vi "Test Control Panel(Blake).vi"() -> ()   [LabVIEW 2017, in "Synapse CCD.lvclass"]
uses:
  Synapse CCD.lvclass
  Areas.ctl
  <vilib>/Utility/error.llb/DialogType.ctl
  Synapse CCD.lvclass/Synapse CCD.ctl
  Spectrometer Triax 550/JY-SPEX-TRIAX/controls.llb/Slits.ctl
  Global/GPIB Numbers.vi
  Spectrometer Triax 550/JY-SPEX-TRIAX/JY-SPEX-TRIAX.lvlib
panel:
  out "laser Pulse":dbl[unit]
  in  "estimate laser Pulse?":bool
  in  "error in (no error)":errorcluster
  out "CCD \nInitialized":bool
  out "JYCCDLib.IJYCCDReqd 1":refnum<k7>
  out "Spectrometer \nInitialized":bool
  in  "File Name":path
  out "error out":errorcluster
  in  "Go to start\nof raster scan":bool
  in  "Raster explanation":bool
  in  "Repeat Capture":bool
  in  "Export\nPlot":bool
  in  "Take Spectrum":bool
  in  "Set CCD":bool
  in  "Set Grating":bool
  in  "Copy Actual to Set":bool
  in  "Populate Fields with Member Data":bool
  in  "Bin width (pixels)":i32=1 min=1 max=1024 step=1
  in  "Number of CCD bins to use each snapshot":i32=1 min=1 max=1024 step=1
  in  "Raster Scan":bool
  in  "Cosmic Ray\nRemoval?":bool
  in  "# to Average":u32=1
  in  "Averaging?":bool
  in  "Time Between Acq. (ms)":u32
  in  "Dark Subtract?":bool
  out "Status":string
  out "Max slit resolution":dbl[unit]
  out "Warning: counts \nwent too high!":bool
  out "Resolution\n(nm/pixel)":dbl[unit] format="%#_3g"
  out "where am i?":string
  out "Total possible CCD bins":dbl=20.48
  out "Cosmic Ray Locations":string
  out "Bin width (nm)\n(scan resolution)":dbl[unit]=3.7e-11
  in  "Start":dbl[unit]
  in  "End":dbl[unit]
  in  "Exit Slit":dbl[unit]
  in  "Entrance Slit":dbl[unit]
  out "Min":dbl[unit]
  out "Max":dbl[unit]
  in  "Center Wavelength":dbl[unit]
  in  "Grating":u16(ring) items=["1200 lines/mm - 500 nm Blaze", "1200 lines/mm - 750 nm Blaze", "600 lines/mm - 1000 nm Blaze"]
  in  "GAIN":u16(ring) caption="Device Name" items=["High Light", "Best Dynamic", "High Sensitivity"]
  in  "ADC":u16(ring) caption="Device Name" items=["   20 kHz", "1 MHz", "1 MHz Ultra"]
  in  "Integration time":dbl[unit]=0.01
  in  "stop":bool
  in  "image mode":bool
  out "Spectrum":cluster{"Ramp Pattern":dbl[], "X array":dbl[]}[](graph)
  out "UnProcessed Spectra":T1(graph)
  out "Max value of last snapshot":i32
  out "populate fields with member data: CCD private data":T3={"JYCCDLib.IJYCCDReqd"=refnum, "JYMONOLib.IJYMonoReqd"=refnum, "Integration time"=0.01, "ADC"=0, "GAIN"=0, "Areas"=[[1, 1, 1, 1024, 256, 1, 256]], "Most Recent Data Object"=refnum, "Mono Properties"={"Grating"=0, "Center Wavelength"=0.0, "Entrance Slit"=0.0, "Exit Slit"=0.0}, "Coverage"={"Max"=0.0, "Min"=0.0}, "Multi-Acquisitions"={"Dark Subtract?"=FALSE, "Averaging?"=FALSE, "Cosmic Ray Removal?"=FALSE, "# to Average"=0, "Time Between Acq."=0, "Acquisitions Control Array"=[TRUE], "Raw Data"=[], "Processed Data"=[], "Array of Wavelengths"=[]}, "Raster Scan"={"Raster Scan?"=FALSE, "Start"=0.0, "End"=0.0, "Bin width (pixels)"=1, "Bin width (nm)\n(scan resolution)"=3.7e-11, "Number of CCD bins to use each snapshot"=1, "Total possible CCD bins"=20.48, "Warning: counts \nwent too high!"=FALSE}} {"Raster Scan"."Number of CCD bins to use each snapshot" min=1 max=1024 step=1; "Raster Scan"."Bin width (pixels)" min=1 max=1024 step=1; "Mono Properties"."Grating" items=["1200 lines/mm - 500 nm Blaze", "1200 lines/mm - 750 nm Blaze", "600 lines/mm - 1000 nm Blaze"]; "GAIN" items=["High Light", "Best Dynamic", "High Sensitivity"]; "ADC" items=["   20 kHz", "1 MHz", "1 MHz Ultra"]}
types:
  T1 = cluster{"Array of Wavelengths":dbl[], "Raw Data":i32[]}[]
  T2 = typedef "Synapse CCD.lvclass/Areas.ctl" = i32[][]
  T3 = cluster{"JYCCDLib.IJYCCDReqd":refnum<k7>, "JYMONOLib.IJYMonoReqd":refnum<k7>, "Integration time":dbl[unit], "ADC":u16, "GAIN":u16, "Areas":T2, "Most Recent Data Object":refnum<k7>, "Mono Properties":cluster{"Grating":u16, "Center Wavelength":dbl[unit], "Entrance Slit":dbl[unit], "Exit Slit":dbl[unit]}, "Coverage":cluster{"Max":dbl[unit], "Min":dbl[unit]}, "Multi-Acquisitions":cluster{"Dark Subtract?":bool, "Averaging?":bool, "Cosmic Ray Removal?":bool, "# to Average":u32, "Time Between Acq.":u32, "Acquisitions Control Array":bool[], "Raw Data":i32[][], "Processed Data":dbl[], "Array of Wavelengths":dbl[]}, "Raster Scan":cluster{"Raster Scan?":bool, "Start":dbl[unit], "End":dbl[unit], "Bin width (pixels)":i32, "Bin width (nm)\n(scan resolution)":dbl[unit], "Number of CCD bins to use each snapshot":i32, "Total possible CCD bins":dbl, "Warning: counts \nwent too high!":bool}}
  T4 = typedef "DialogType.ctl" = u16
  T5 = typedef "GPIB Type Def.ctl" = cluster{"Name":string, "bus":dbl, "GPIB":dbl, "GPIB as string":string, "byte":i32, "VISA Resource Name":refnum<visa-resource-name>}
  T6 = typedef "JY-SPEX-TRIAX.lvlib/Slits.ctl" = enum16{"0 (Front/Axial Entrance)", "1 (Side/Lateral Entrance)", "2 (Front/Axial Exit)", "3 (Side/Lateral Exit)"}
  T7 = cluster{"Grating":u16, "Center Wavelength":dbl[unit], "Entrance Slit":dbl[unit], "Exit Slit":dbl[unit]}
  T8 = cluster{"Dark Subtract?":bool, "Averaging?":bool, "Cosmic Ray Removal?":bool, "# to Average":u32, "Time Between Acq.":u32, "Acquisitions Control Array":bool[], "Raw Data":i32[][], "Processed Data":dbl[], "Array of Wavelengths":dbl[]}
  T9 = cluster{"Raster Scan?":bool, "Start":dbl[unit], "End":dbl[unit], "Bin width (pixels)":i32, "Bin width (nm)\n(scan resolution)":dbl[unit], "Number of CCD bins to use each snapshot":i32, "Total possible CCD bins":dbl, "Warning: counts \nwent too high!":bool}
  T10 = cluster{"Array of Wavelengths":dbl[], "Raw Data":i32[]}
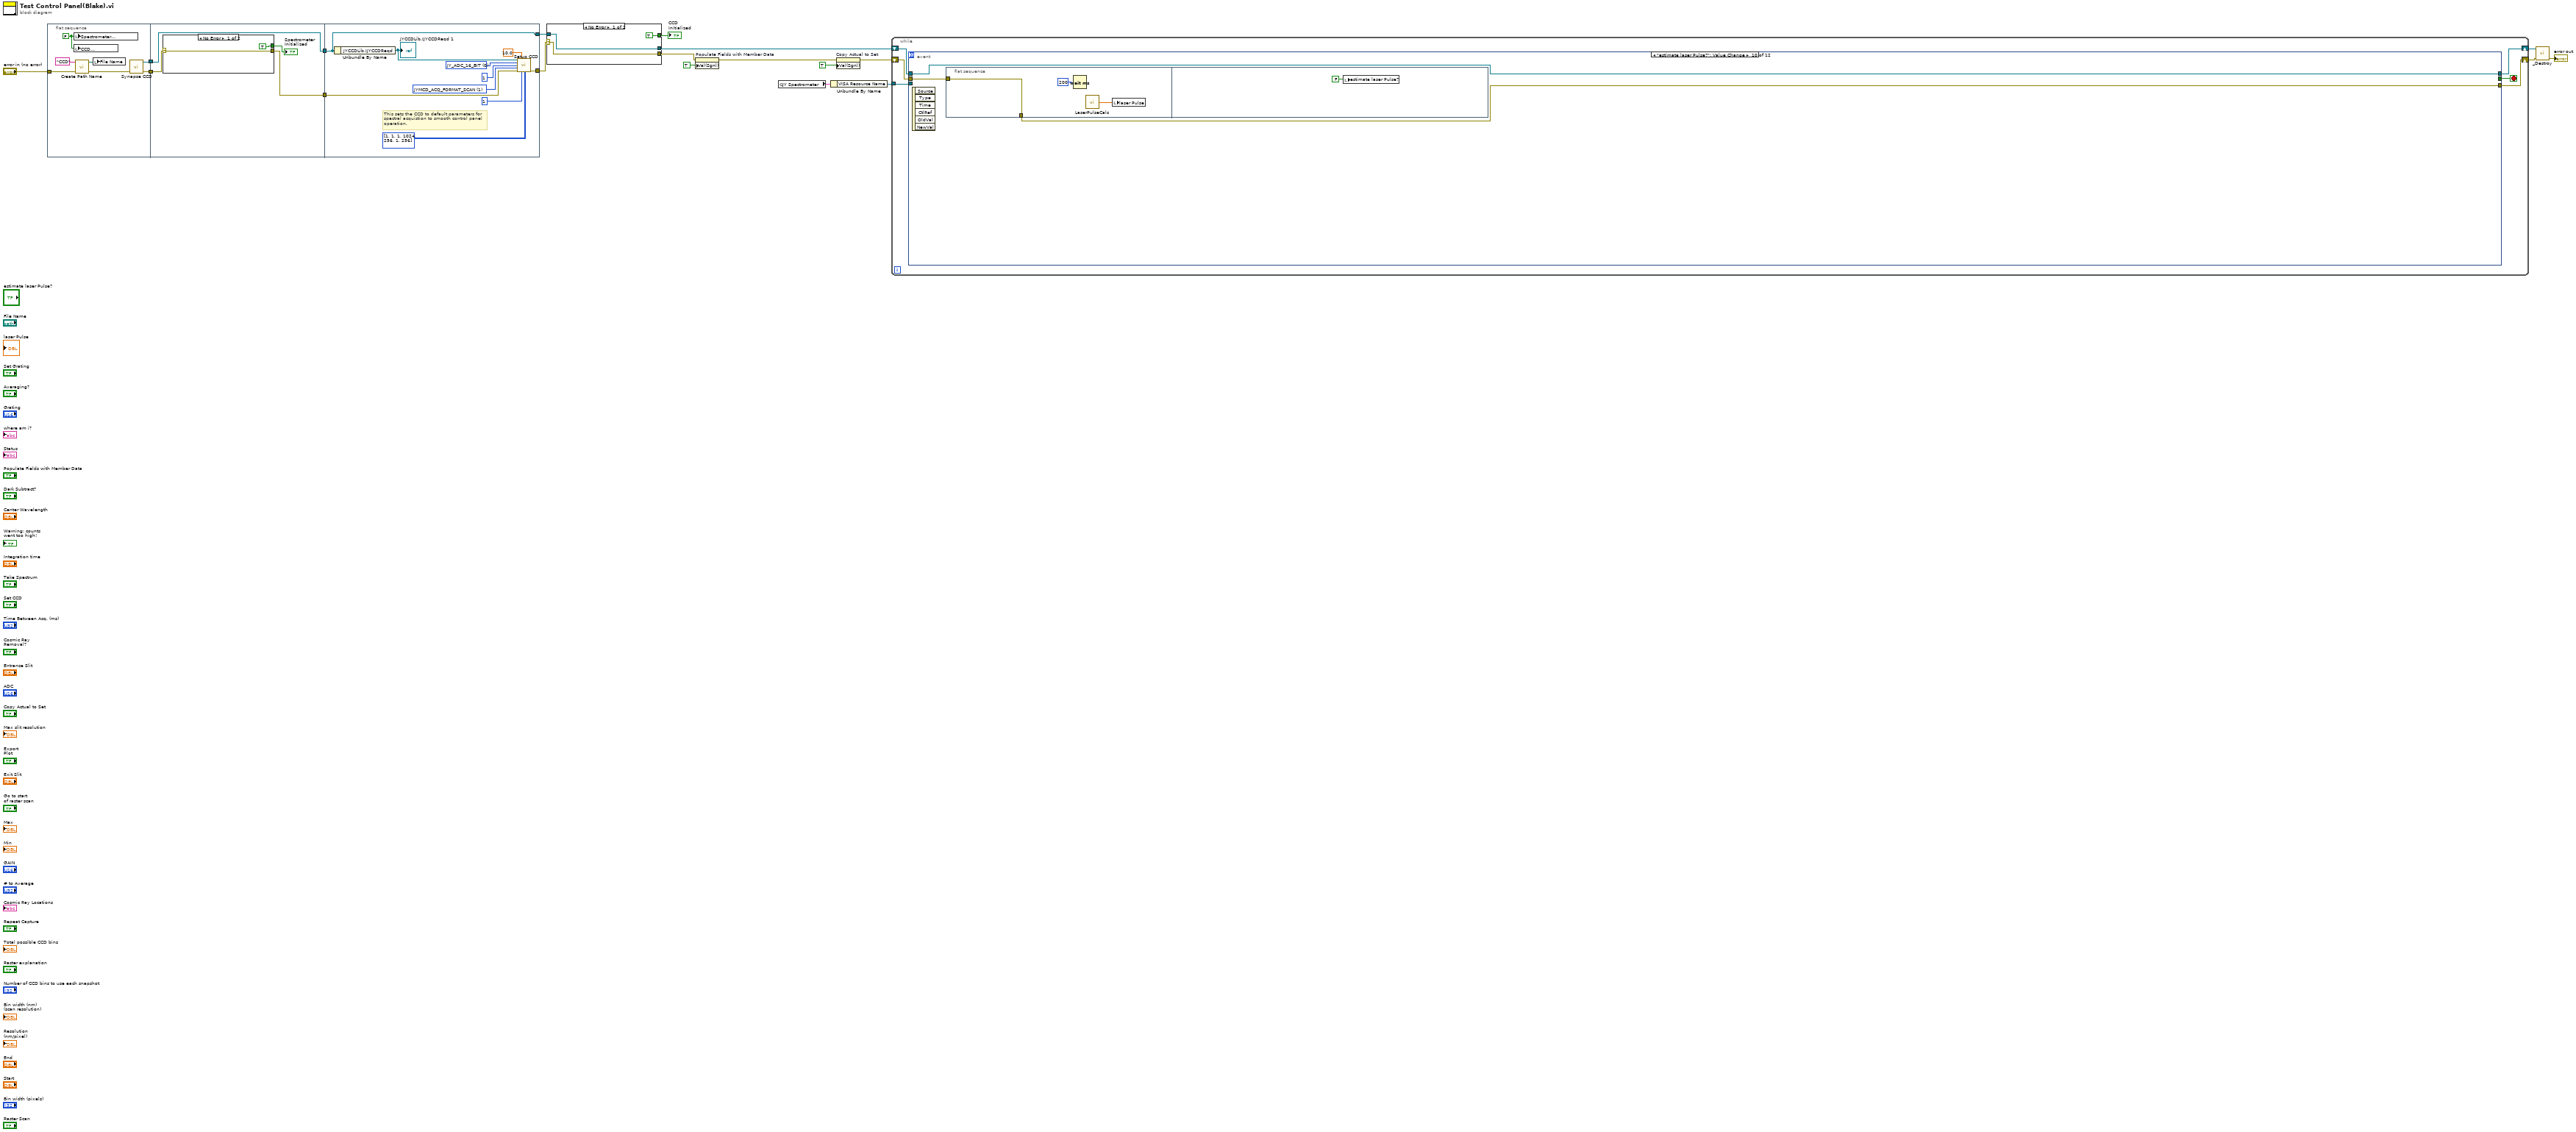
[diagram p0: block diagram]
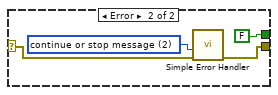
[diagram p2: hidden frame]
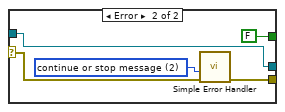
[diagram p3: hidden frame]
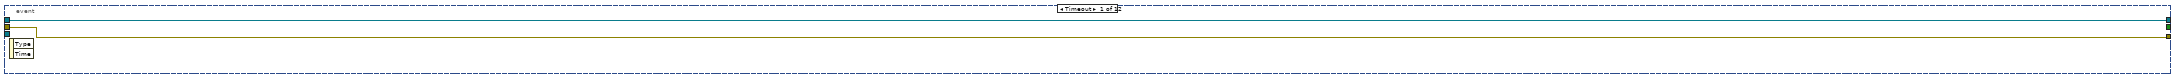
[diagram p4: hidden frame]
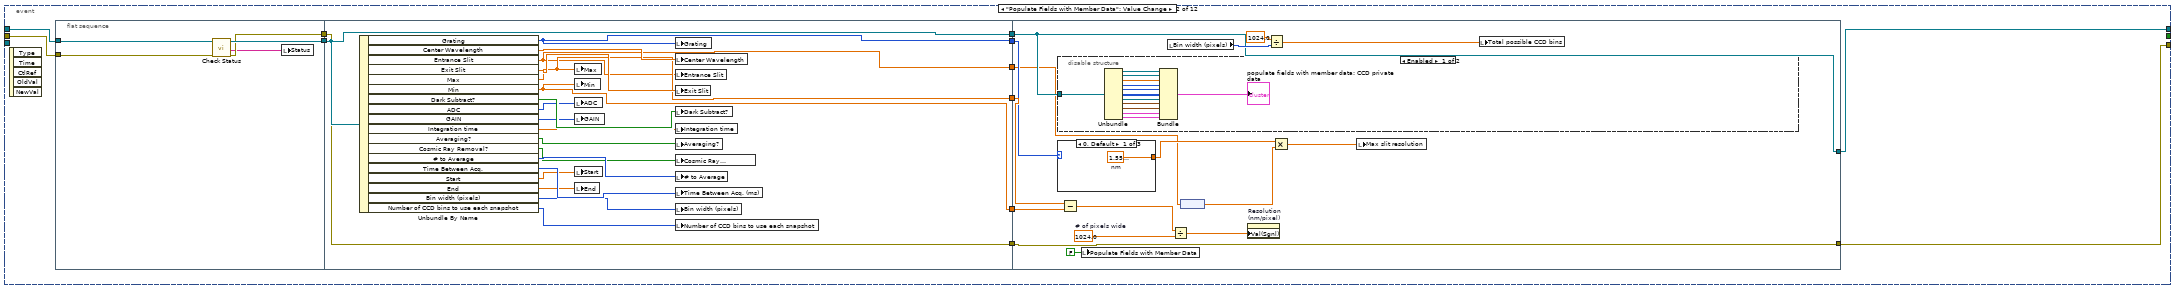
[diagram p5: hidden frame]
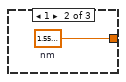
[diagram p6: hidden frame]
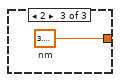
[diagram p7: hidden frame]
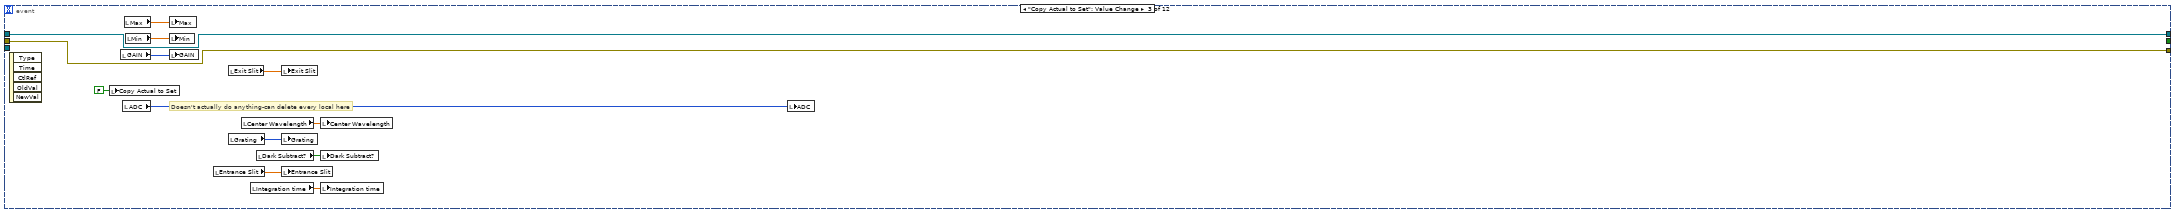
[diagram p9: hidden frame]
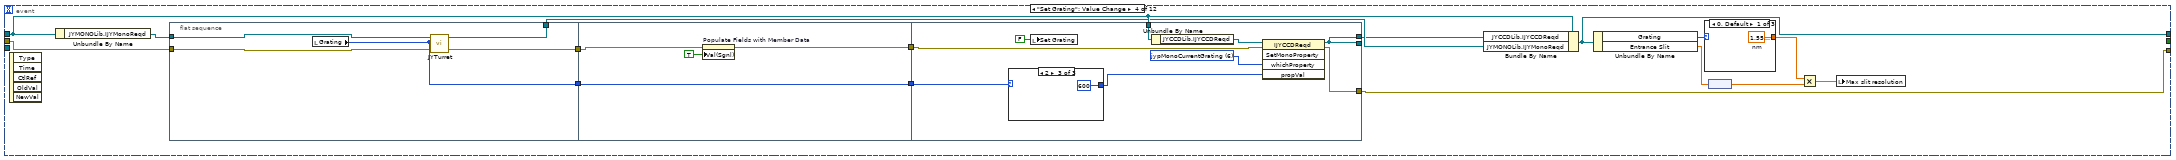
[diagram p10: hidden frame]
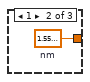
[diagram p11: hidden frame]
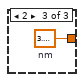
[diagram p12: hidden frame]
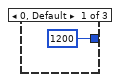
[diagram p13: hidden frame]
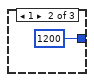
[diagram p14: hidden frame]
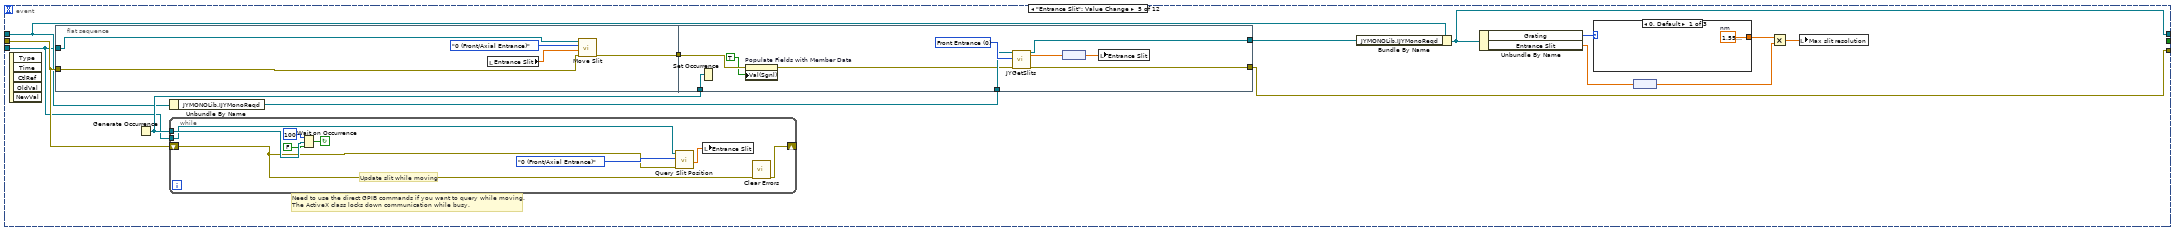
[diagram p15: hidden frame]
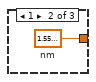
[diagram p16: hidden frame]
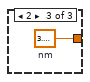
[diagram p17: hidden frame]
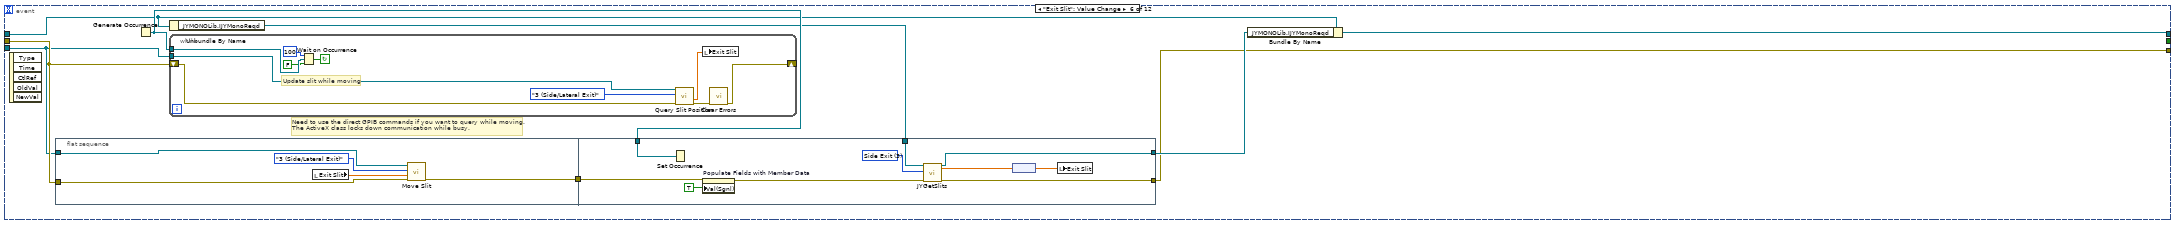
[diagram p18: hidden frame]
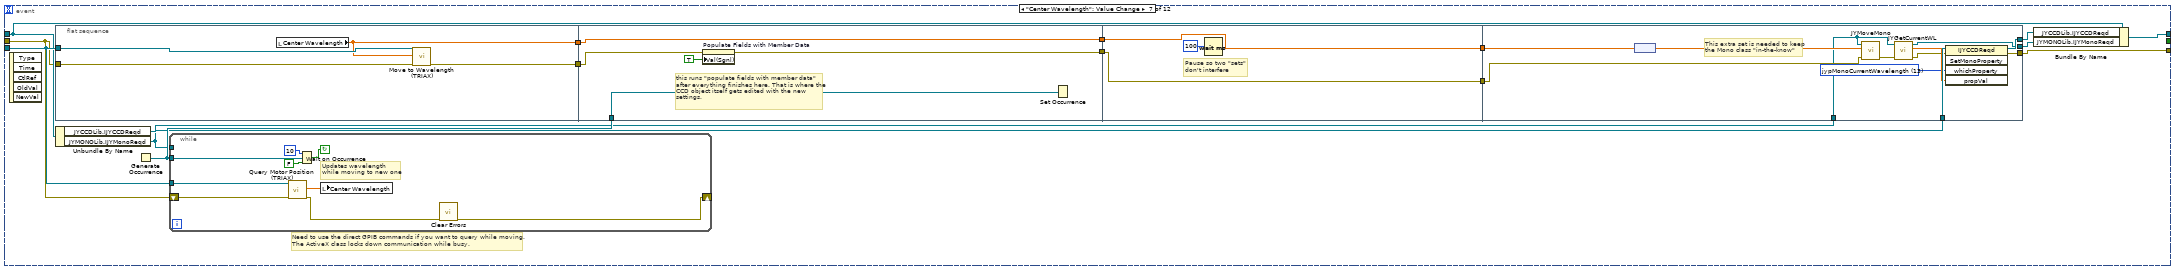
[diagram p19: hidden frame]
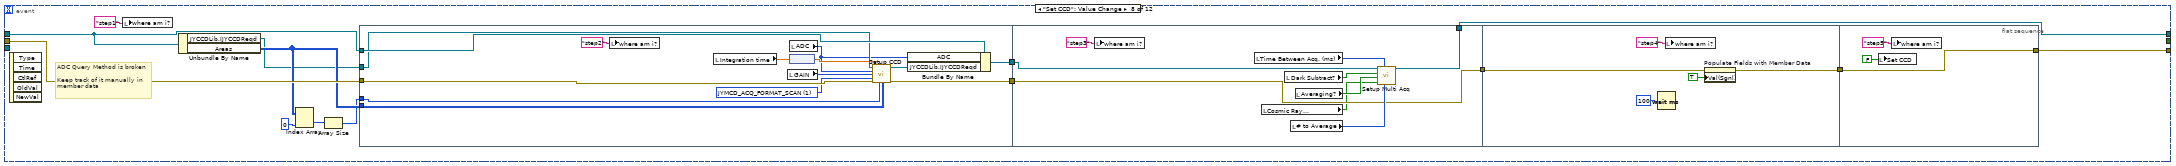
[diagram p20: hidden frame]
diagram:
  n1 = flat-sequence {
    tunnel: "error in (no error)" -> [w24]
    tunnel: [w26] -> w16
    tunnel: [w25] -> w15
    tunnel: w16 -> [w30]
    tunnel: [w29] -> w14
    tunnel: w15 -> [w27]
    tunnel: [w27] -> w13
    tunnel: [w46] -> w9
    tunnel: [w37] -> w12
    tunnel: w14 -> [w40]
    tunnel: w13 -> [w46]
    frame #0 {
      w20 = FALSE ("Spectrometer Initialized")
      n2 = local write "Spectrometer \nInitialized"(w20) -> ()
      n3 = local write "CCD \nInitialized"(w20) -> ()
      n4 = call "Create Path Name.vi"("error in"=w24, "filename"="CCD") -> ("error out"=w23:errorcluster, "path"=w21:path)  [unwired: 1 in, 3 out]
      n5 = local write "File Name"(w21) -> ()
      n6 = call "Synapse CCD.vi"("error in (no error)"=w23) -> ("error out"=w26:errorcluster, "Synapse CCD.lvclass"=w25:refnum<class "Synapse CCD.lvclass">)  [unwired: 9 in]
    }
    frame #1 {
      n7 = case shown="No Error" w30 {
        selector: w30 -> [w32 w35]
        tunnel: [w32 w34] -> w29
        tunnel: [TRUE FALSE] -> w28
        frame No Error {
        }
        frame Error {
          w33 = T4 2 items=["no dialog", "OK message", "continue or stop message", "OK message + warnings", "continue/stop + warnings"] ("type of dialog (OK msg:1)")
          n8 = call <vilib>:"Simple Error Handler.vi"("type of dialog (OK msg:1)"=w33, "error in (no error)"=w35) -> ("error out"=w34:errorcluster)  [unwired: 3 in, 4 out]
        }
      }
      "Spectrometer \nInitialized" <- w28
    }
    frame #2 {
      w41 = 1 items=["JYMCD_ACQ_FORMAT_IMAGE", "JYMCD_ACQ_FORMAT_SCAN"] ("Acquisition type")
      w43 = 0 items=["JY_ADC_16_BIT", "JY_ADC_14_BIT", "JY_ADC_18_BIT"] ("Select ADC")
      # "This sets the CCD to default parameters for\nspectral acquistion to smooth control panel\noperation."
      n9 = Unbundle By Name(w46) -> ("JYCCDLib.IJYCCDReqd"=w45:refnum<k7>)
      "JYCCDLib.IJYCCDReqd 1" <- w45
      n10 = call "Setup CCD.vi"("IJYCCDReqd In"=w45, "Integration time(ms)"=10.0 ("IntegrationTime"), "Select ADC"=w43, "Gain"=1, "Acquisition type"=w41, "error in (no error)"=w40, "numAreas"=1, "areas :"=T2 [[1, 1, 1, 1024, 256, 1, 256]] ("Areas")) -> ("error out"=w37:errorcluster)  [unwired: 5 in, 2 out]
    }
  }
  n11 = case shown="No Error" w12 {
    selector: w12 -> [w48 w53]
    tunnel: w9 -> [w49 w54]
    tunnel: [w49 w54] -> w7
    tunnel: [w48 w52] -> w5
    tunnel: [TRUE FALSE] -> w10
    frame No Error {
    }
    frame Error {
      w51 = T4 2 items=["no dialog", "OK message", "continue or stop message", "OK message + warnings", "continue/stop + warnings"] ("type of dialog (OK msg:1)")
      n12 = call <vilib>:"Simple Error Handler.vi"("type of dialog (OK msg:1)"=w51, "error in (no error)"=w53) -> ("error out"=w52:errorcluster)  [unwired: 3 in, 4 out]
    }
  }
  "CCD \nInitialized" <- w10
  n13 = property on="Populate Fields with Member Data" class="Bool (strict)"(error in=w5, "Val(Sgnl)"=TRUE ("Value (Signaling)")) -> (error out=w3:errorcluster)  [unwired: 1 in, 1 out]
  n14 = global read "GPIB Numbers.vi" "JY Spectrometer"() -> (w11:T5)
  n15 = Unbundle By Name(w11) -> ("VISA Resource Name"=w8:refnum<visa-resource-name>)
  n16 = property on="Copy Actual to Set" class="Bool (strict)"(error in=w3, "Val(Sgnl)"=TRUE ("Value (Signaling)")) -> (error out=w1:errorcluster)  [unwired: 1 in, 1 out]
  n17 = while {
    shift-right: [w55] -> w17
    shift-left: w1 -> [w59]
    shift-right: [w56] -> w18
    shift-left: w7 -> [w60]
    tunnel: w8 -> [w58]
    stop <- w57 stop-if-true
    n18 = event shown="[9] \"estimate laser Pulse?\": Value Change" {
      selector: _ -> [_ _ _ _ _ _ _ _ _ _ _ _]
      dyn-events: _ -> [_ _ _ _ _ _ _ _ _ _ _ _]
      timeout: _ -> [_ _ _ _ _ _ _ _ _ _ _ _]
      tunnel: w60 -> [w62 w67 w133 w154 w194 w228 w272 w314 w359 w392 _ w401]
      tunnel: w59 -> [w61 w74 w132 w156 w197 w232 w264 w322 w360 w393 _ w402]
      tunnel: [w61 w65 w132 w151 w191 w227 w263 w313 w354 w394 _ w402] -> w55
      tunnel: [w62 w66 w133 w148 w188 w226 w262 w312 w363 w392 _ w401] -> w56
      tunnel: [_ _ _ _ _ _ _ _ _ _ _ "stop"] -> w57
      tunnel: w58 -> [_ _ _ _ w193 w230 w273 _ _ _ _ _]
      event Timeout {
        n19 = event-data() -> ()  [unwired: 1 in, 2 out]
      }
      event "Populate Fields with Member Data": Value Change {
        n20 = event-data() -> ()  [unwired: 1 in, 5 out]
        n21 = flat-sequence {
          tunnel: w74 -> [w77]
          tunnel: w67 -> [w79]
          tunnel: [w78] -> w71
          tunnel: [w76] -> w70
          tunnel: [w93] -> w73
          tunnel: [w86] -> w72
          tunnel: w71 -> [w93]
          tunnel: w70 -> [w86]
          tunnel: [w88] -> w69
          tunnel: [w87] -> w68
          tunnel: [w85] -> w64
          tunnel: [w84] -> w63
          tunnel: [w115] -> w65
          tunnel: [w106] -> w66
          tunnel: w73 -> [w106]
          tunnel: w72 -> [w115]
          tunnel: w69 -> [w110]
          tunnel: w68 -> [w111]
          tunnel: w64 -> [w104]
          tunnel: w63 -> [w101]
          frame #0 {
            n22 = call-dynamic "Check Status.vi"("error in (no error)"=w77, "Synapse CCD in"=w79) -> ("error out"=w76:errorcluster, "Status"=w75:string, "Synapse CCD out"=w78:refnum<class "Synapse CCD.lvclass">)  [unwired: 6 in, 1 out]
            n23 = local write "Status"(w75) -> ()
          }
          frame #1 {
            n24 = Unbundle By Name(w93) -> ("Grating"=w85:u16, "Center Wavelength"=w99:dbl[unit], "Entrance Slit"=w84:dbl[unit], "Exit Slit"=w98:dbl[unit], "Max"=w88:dbl[unit], "Min"=w87:dbl[unit], "Dark Subtract?"=w97:bool, "ADC"=w96:u16, "GAIN"=w95:u16, "Integration time"=w94:dbl[unit], "Averaging?"=w89:bool, "Cosmic Ray Removal?"=w90:bool, "# to Average"=w91:u32, "Time Between Acq."=w92:u32, "Start"=w83:dbl[unit], "End"=w82:dbl[unit], "Bin width (pixels)"=w81:i32, "Number of CCD bins to use each snapshot"=w80:i32)
            n25 = local write "Max"(w88) -> ()
            n26 = local write "Min"(w87) -> ()
            n27 = local write "ADC"(w96) -> ()
            n28 = local write "GAIN"(w95) -> ()
            n29 = local write "Start"(w83) -> ()
            n30 = local write "End"(w82) -> ()
            n31 = local write "Grating"(w85) -> ()
            n32 = local write "Center Wavelength"(w99) -> ()
            n33 = local write "Entrance Slit"(w84) -> ()
            n34 = local write "Exit Slit"(w98) -> ()
            n35 = local write "Dark Subtract?"(w97) -> ()
            n36 = local write "Integration time"(w94) -> ()
            n37 = local write "Averaging?"(w89) -> ()
            n38 = local write "Cosmic Ray\nRemoval?"(w90) -> ()
            n39 = local write "# to Average"(w91) -> ()
            n40 = local write "Time Between Acq. (ms)"(w92) -> ()
            n41 = local write "Bin width (pixels)"(w81) -> ()
            n42 = local write "Number of CCD bins to use each snapshot"(w80) -> ()
          }
          frame #2 {
            w112 = 1024.0  # # of pixels wide
            n43 = disable-structure shown="Enabled" {
              disable-tunnel: w106 -> [w123 _]
              frame Enabled {
                n44 = Unbundle(w123) -> (w131:refnum<k7>, w130:refnum<k7>, w129:dbl[unit], w128:u16, w127:u16, w126:T2, w125:refnum<k7>, w124:T7, w122:cluster{"Max":dbl[unit], "Min":dbl[unit]}, w121:T8, w120:T9)
                n45 = Bundle("JYCCDLib.IJYCCDReqd"=w131, "JYMONOLib.IJYMonoReqd"=w130, "Integration time"=w129, "ADC"=w128, "GAIN"=w127, "Areas"=w126, "Most Recent Data Object"=w125, "Mono Properties"=w124, "Coverage"=w122, "Multi-Acquisitions"=w121, "Raster Scan"=w120) -> (→"populate fields with member data: CCD private data":T3)  [unwired: 1 in]
              }
              frame Disabled {
              }
            }
            n46 = case shown="0, Default" w104 {
              tunnel: [w116 w117 w118] -> w103
              frame 0, Default {
                w116 = dbl[unit] 1.5500000000000002e-09  # nm
              }
              frame 1 {
                w117 = dbl[unit] 1.5500000000000002e-09  # nm
              }
              frame 2 {
                w118 = dbl[unit] 3.1000000000000005e-09  # nm
              }
            }
            n47 = Subtract(x=w110, y=w111) -> (x-y=w113:dbl[unit])
            n48 = local write "Populate Fields with Member Data"(FALSE ("Populate Fields with Member Data")) -> ()
            n49 = local read "Bin width (pixels)"() -> (w108:i32)
            n50 = Divide(x=w113, y=w112) -> (x/y=w105:dbl[unit])
            n51 = node(w101) -> (w100:dbl)
            n52 = property on="Resolution\n(nm/pixel)" class="DigNum (strict)"("Val(Sgnl)"=w105) -> ()  [unwired: 2 in, 2 out]
            n53 = Divide(x=1024.0, y=w108) -> (x/y=w109:dbl)
            n54 = Multiply(x=w103, y=w100) -> (x*y=w102:dbl[unit])
            n55 = local write "Max slit resolution"(w102) -> ()
            n56 = local write "Total possible CCD bins"(w109) -> ()
          }
        }
      }
      event "Copy Actual to Set": Value Change {
        # "Doesn't actually do anything-can delete every local here"
        n57 = event-data() -> ()  [unwired: 1 in, 5 out]
        n58 = local write "Copy Actual to Set"(FALSE ("Copy Actual to Set")) -> ()
        n59 = local read "GAIN"() -> (w138:u16)
        n60 = local read "ADC"() -> (w144:u16)
        n61 = local read "Max"() -> (w135:dbl[unit])
        n62 = local read "Min"() -> (w141:dbl[unit])
        n63 = local write "Max"(w135) -> ()
        n64 = local write "Min"(w141) -> ()
        n65 = local write "GAIN"(w138) -> ()
        n66 = local read "Entrance Slit"() -> (w140:dbl[unit])
        n67 = local read "Exit Slit"() -> (w139:dbl[unit])
        n68 = local read "Grating"() -> (w137:u16)
        n69 = local read "Center Wavelength"() -> (w143:dbl[unit])
        n70 = local read "Integration time"() -> (w136:dbl[unit])
        n71 = local read "Dark Subtract?"() -> (w142:bool)
        n72 = local write "Exit Slit"(w139) -> ()
        n73 = local write "Grating"(w137) -> ()
        n74 = local write "Entrance Slit"(w140) -> ()
        n75 = local write "Center Wavelength"(w143) -> ()
        n76 = local write "Dark Subtract?"(w142) -> ()
        n77 = local write "Integration time"(w136) -> ()
        n78 = local write "ADC"(w144) -> ()
      }
      event "Set Grating": Value Change {
        n79 = event-data() -> ()  [unwired: 1 in, 5 out]
        n80 = Unbundle By Name(w154) -> ("JYMONOLib.IJYMonoReqd"=w155:refnum<k7>)
        n81 = flat-sequence {
          tunnel: w155 -> [w166]
          tunnel: w156 -> [w167]
          tunnel: [w164] -> w160
          tunnel: [w168] -> w158
          tunnel: [w165] -> w153
          tunnel: w160 -> [w172]
          tunnel: [w171] -> w159
          tunnel: w158 -> [w171]
          tunnel: [w169] -> w157
          tunnel: [w174] -> w151
          tunnel: w159 -> [w180]
          tunnel: w157 -> [w177]
          tunnel: [w173] -> _
          tunnel: w154 -> [w179]
          tunnel: [w173] -> w152
          frame #0 {
            n82 = local read "Grating"() -> (w168:u16)
            n83 = call "JYTurret.vi"("error in (no error)"=w167, "Grating Index"=w168, "JYMONOLib.IJYMonoReqd In"=w166) -> ("error out"=w164:errorcluster, "JYMONOLib.IJYMonoReqd Out"=w165:refnum<k7>)  [unwired: 1 out]
          }
          frame #1 {
            n84 = property on="Populate Fields with Member Data" class="Bool (strict)"(error in=w172, "Val(Sgnl)"=TRUE ("Value (Signaling)")) -> (error out=w169:errorcluster)  [unwired: 1 in, 1 out]
          }
          frame #2 {
            w178 = 6 items=["jyUndefined", "jypMonoLinearDispersion", "jypMonoBacklashAmount", "jypMonoStepsPerUnit", "jypMonoBaseUnits", "jypMonoBaseGrating", "jypMonoCurrentGrating", "jypMonoMaxLimit", "jypMonoMinLimit", "jypMonoTiltAngle", "jypMonoIncludedAngle", "jypMonoFocalLength", "jypMonoOrder", "jypMonoCurrentWavelength", "jypMonoMCDWavelengthDirection", "jypBandpassUnits", "jypSlitMaxLimit", "jypSlitMinLimit", "jypSlitBackLashAmount", "jypSlitBaseUnits", "jypSlitStepsPerUnit", "jypLaserLine", "jypTotalHardwarePropertiesPlusOne", "jypCurrentTurretPosition"] ("whichProperty")
            n85 = case shown="2" w180 {
              tunnel: [u16 1200 u16 1200 u16 600] -> w175
              frame 0, Default {
              }
              frame 1 {
              }
              frame 2 {
              }
            }
            n86 = local write "Set Grating"(FALSE ("Set Spectrometer")) -> ()
            n87 = Unbundle By Name(w179) -> ("JYCCDLib.IJYCCDReqd"=w176:refnum<k7>)
            n88 = invoke class="IJYCCDReqd" method="SetMonoProperty"(reference=w176, error in=w177, "whichProperty"=w178, "propVal"=w175) -> (reference out=w173:refnum<k7>, error out=w174:errorcluster)  [unwired: 1 in, 3 out]
          }
        }
        n89 = Bundle By Name(cluster=w154, "JYCCDLib.IJYCCDReqd"=w152, "JYMONOLib.IJYMonoReqd"=w153) -> (w148:refnum<class "Synapse CCD.lvclass">)
        n90 = Unbundle By Name(w148) -> ("Grating"=w147:u16, "Entrance Slit"=w146:dbl[unit])
        n91 = case shown="0, Default" w147 {
          tunnel: [w161 w162 w163] -> w150
          frame 0, Default {
            w161 = dbl[unit] 1.5500000000000002e-09  # nm
          }
          frame 1 {
            w162 = dbl[unit] 1.5500000000000002e-09  # nm
          }
          frame 2 {
            w163 = dbl[unit] 3.1000000000000005e-09  # nm
          }
        }
        n92 = node(w146) -> (w149:dbl)
        n93 = Multiply(x=w150, y=w149) -> (x*y=w145:dbl[unit])
        n94 = local write "Max slit resolution"(w145) -> ()
      }
      event "Entrance Slit": Value Change {
        # "Need to use the direct GPIB commands if you want to query while moving.\nThe ActiveX class locks down communication while busy."
        n95 = event-data() -> ()  [unwired: 1 in, 5 out]
        n96 = flat-sequence {
          tunnel: w197 -> [w212]
          tunnel: [w215] -> w198
          tunnel: w193 -> [w213]
          tunnel: w198 -> [w220]
          tunnel: [w216] -> w191
          tunnel: w196 -> [w225]
          tunnel: w195 -> [w223]
          tunnel: [w221] -> w192
          frame #0 {
            n97 = local read "Entrance Slit"() -> (w211:dbl[unit])
            n98 = call "Move Slit.vi"("error in (no error)"=w212, "Desired Slit Position"=w211, "Slit (Front/Axial Entrance)"=Slits."0 (Front/Axial Entrance)", "VISA resource name"=w213) -> ("error out"=w215:errorcluster)  [unwired: 6 in, 1 out]
          }
          frame #1 {
            w224 = u16 0 items=["Front Entrance", "Side Entrance", "Front Exit", "Side Exit", "First Intermediate", "Second Intermediate"] ("Slit")
            n99 = Set Occurrence(w225) -> ()
            n100 = property on="Populate Fields with Member Data" class="Bool (strict)"(error in=w220, "Val(Sgnl)"=TRUE ("Value (Signaling)")) -> (error out=w218:errorcluster)  [unwired: 1 in, 1 out]
            n101 = call "JYGetSlits.vi"("MonoRefNum IN"=w223, "Slit"=w224, "error in (no error)"=w218) -> ("MonoRefNum Out"=w221:refnum<k7>, "Slit Width"=w217:dbl, "error out"=w216:errorcluster)  [unwired: 13 in, 1 out]
            n102 = node(w217) -> (w222:dbl[unit])
            n103 = local write "Entrance Slit"(w222) -> ()
          }
        }
        n104 = Generate Occurrence() -> (w196:refnum<k4>)
        n105 = Unbundle By Name(w194) -> ("JYMONOLib.IJYMonoReqd"=w195:refnum<k7>)
        n106 = while {
          tunnel: w196 -> [w210]
          shift-right: [w202] -> _
          shift-left: w197 -> [w203]
          tunnel: w193 -> [w206]
          stop <- w209 continue-if-true
          # "Update slit while moving"
          n107 = Wait on Occurrence(1:FALSE ("ignore previous (T)"), 2:w210, 3:100 ("ms timeout (-1)")) -> (0:w209:bool)
          n108 = call "Query Slit Position.vi"("error in (no error)"=w203, "Slit (Front/Axial Entrance)"=Slits."0 (Front/Axial Entrance)", "VISA resource name"=w206) -> ("Slit Position"=w204:dbl[unit])  [unwired: 6 in, 2 out]
          n109 = local write "Entrance Slit"(w204) -> ()
          n110 = call <vilib>:"Clear Errors.vi"("error in (no error)"=w203) -> ("error out"=w202:errorcluster)  [unwired: 5 in, 1 out]
        }
        n111 = Bundle By Name(cluster=w194, "JYMONOLib.IJYMonoReqd"=w192) -> (w188:refnum<class "Synapse CCD.lvclass">)
        n112 = Unbundle By Name(w188) -> ("Grating"=w187:u16, "Entrance Slit"=w186:dbl[unit])
        n113 = case shown="0, Default" w187 {
          tunnel: [w199 w200 w201] -> w190
          frame 0, Default {
            w199 = dbl[unit] 1.5500000000000002e-09  # nm
          }
          frame 1 {
            w200 = dbl[unit] 1.5500000000000002e-09  # nm
          }
          frame 2 {
            w201 = dbl[unit] 3.1000000000000005e-09  # nm
          }
        }
        n114 = node(w186) -> (w189:dbl)
        n115 = Multiply(x=w190, y=w189) -> (x*y=w185:dbl[unit])
        n116 = local write "Max slit resolution"(w185) -> ()
      }
      event "Exit Slit": Value Change {
        # "Need to use the direct GPIB commands if you want to query while moving.\nThe ActiveX class locks down communication while busy."
        n117 = event-data() -> ()  [unwired: 1 in, 5 out]
        n118 = flat-sequence {
          tunnel: w232 -> [w248]
          tunnel: [w245] -> w234
          tunnel: w230 -> [w247]
          tunnel: w234 -> [w253]
          tunnel: [w250] -> w227
          tunnel: w233 -> [w258]
          tunnel: w231 -> [w257]
          tunnel: [w254] -> w229
          frame #0 {
            n119 = local read "Exit Slit"() -> (w246:dbl[unit])
            n120 = call "Move Slit.vi"("error in (no error)"=w248, "Desired Slit Position"=w246, "Slit (Front/Axial Entrance)"=Slits."3 (Side/Lateral Exit)", "VISA resource name"=w247) -> ("error out"=w245:errorcluster)  [unwired: 6 in, 1 out]
          }
          frame #1 {
            w256 = u16 3 items=["Front Entrance", "Side Entrance", "Front Exit", "Side Exit", "First Intermediate", "Second Intermediate"] ("Slit")
            n121 = Set Occurrence(w258) -> ()
            n122 = property on="Populate Fields with Member Data" class="Bool (strict)"(error in=w253, "Val(Sgnl)"=TRUE ("Value (Signaling)")) -> (error out=w252:errorcluster)  [unwired: 1 in, 1 out]
            n123 = call "JYGetSlits.vi"("MonoRefNum IN"=w257, "Slit"=w256, "error in (no error)"=w252) -> ("MonoRefNum Out"=w254:refnum<k7>, "Slit Width"=w251:dbl, "error out"=w250:errorcluster)  [unwired: 13 in, 1 out]
            n124 = node(w251) -> (w255:dbl[unit])
            n125 = local write "Exit Slit"(w255) -> ()
          }
        }
        n126 = Generate Occurrence() -> (w233:refnum<k4>)
        n127 = Unbundle By Name(w228) -> ("JYMONOLib.IJYMonoReqd"=w231:refnum<k7>)
        n128 = while {
          tunnel: w233 -> [w244]
          shift-right: [w235] -> _
          shift-left: w232 -> [w239]
          tunnel: w230 -> [w238]
          stop <- w242 continue-if-true
          # "Update slit while moving"
          n129 = Wait on Occurrence(1:FALSE ("ignore previous (T)"), 2:w244, 3:100 ("ms timeout (-1)")) -> (0:w242:bool)
          n130 = call "Query Slit Position.vi"("error in (no error)"=w239, "Slit (Front/Axial Entrance)"=Slits."3 (Side/Lateral Exit)", "VISA resource name"=w238) -> ("error out"=w236:errorcluster, "Slit Position"=w240:dbl[unit])  [unwired: 6 in, 1 out]
          n131 = local write "Exit Slit"(w240) -> ()
          n132 = call <vilib>:"Clear Errors.vi"("error in (no error)"=w236) -> ("error out"=w235:errorcluster)  [unwired: 5 in, 1 out]
        }
        n133 = Bundle By Name(cluster=w228, "JYMONOLib.IJYMonoReqd"=w229) -> (w226:refnum<class "Synapse CCD.lvclass">)
      }
      event "Center Wavelength": Value Change {
        # "Need to use the direct GPIB commands if you want to query while moving.\nThe ActiveX class locks down communication while busy."
        n134 = event-data() -> ()  [unwired: 1 in, 5 out]
        n135 = flat-sequence {
          tunnel: w264 -> [w288]
          tunnel: [w287] -> w275
          tunnel: w273 -> [w286]
          tunnel: [w285] -> w269
          tunnel: w275 -> [w292]
          tunnel: [w291] -> w268
          tunnel: w274 -> [w289]
          tunnel: [w290] -> w266
          tunnel: w269 -> [w290]
          tunnel: w268 -> [w296]
          tunnel: [w296] -> w267
          tunnel: w266 -> [w295]
          tunnel: [w295] -> w265
          tunnel: [w308] -> w263
          tunnel: w267 -> [w301]
          tunnel: w261 -> [w307]
          tunnel: [w304] -> w271
          tunnel: [w298] -> w270
          tunnel: w265 -> [w302]
          tunnel: w260 -> [w297]
          frame #0 {
            n136 = local read "Center Wavelength"() -> (w285:dbl[unit])
            n137 = call "Move to Wavelength (TRIAX).vi"("error in (no error)"=w288, "Target wavelength"=w285, "VISA resource name"=w286) -> ("error out"=w287:errorcluster)  [unwired: 7 in, 1 out]
          }
          frame #1 {
            # "this runs \"populate fields with member data\" \nafter everything finishes here. That is where the \nCCD object itself gets edited with the new \nsettings."
            n138 = property on="Populate Fields with Member Data" class="Bool (strict)"(error in=w292, "Val(Sgnl)"=TRUE ("Value (Signaling)")) -> (error out=w291:errorcluster)  [unwired: 1 in, 1 out]
            n139 = Set Occurrence(w289) -> ()
          }
          frame #2 {
            # "Pause so two \"sets\" \ndon't interfere"
            n140 = Wait (ms)(milliseconds to wait=u32 100) -> ()  [unwired: 1 out]
          }
          frame #3 {
            w299 = 13 items=["jyUndefined", "jypMonoLinearDispersion", "jypMonoBacklashAmount", "jypMonoStepsPerUnit", "jypMonoBaseUnits", "jypMonoBaseGrating", "jypMonoCurrentGrating", "jypMonoMaxLimit", "jypMonoMinLimit", "jypMonoTiltAngle", "jypMonoIncludedAngle", "jypMonoFocalLength", "jypMonoOrder", "jypMonoCurrentWavelength", "jypMonoMCDWavelengthDirection", "jypBandpassUnits", "jypSlitMaxLimit", "jypSlitMinLimit", "jypSlitBackLashAmount", "jypSlitBaseUnits", "jypSlitStepsPerUnit", "jypLaserLine", "jypTotalHardwarePropertiesPlusOne", "jypCurrentTurretPosition"] ("whichProperty")
            # "This extra set is needed to keep \nthe Mono class \"in-the-know\""
            n141 = node(w302) -> (w300:dbl)
            n142 = call "JYMoveMono.vi"("error in (no error)"=w301, 10:w300, "JYMONOLib.IJYMonoReqd"=w297) -> ("error out"=w303:errorcluster)  [unwired: 8 in]
            n143 = call "JYGetCurrentWL.vi"("error in (no error)"=w303, "JYMONOLib.IJYMonoReqd In"=w297) -> ("error out"=w305:errorcluster, "Current WL"=w306:dbl, "JYMONOLib.IJYMonoReqd Out"=w298:refnum<k7>)  [unwired: 6 in, 1 out]
            n144 = invoke class="IJYCCDReqd" method="SetMonoProperty"(reference=w307, error in=w305, "whichProperty"=w299, "propVal"=w306) -> (reference out=w304:refnum<k7>, error out=w308:errorcluster)  [unwired: 1 in, 3 out]
          }
        }
        n145 = Unbundle By Name(w272) -> ("JYCCDLib.IJYCCDReqd"=w261:refnum<k7>, "JYMONOLib.IJYMonoReqd"=w260:refnum<k7>)
        n146 = Generate Occurrence() -> (w274:refnum<k4>)
        n147 = while {
          tunnel: w274 -> [w284]
          tunnel: w260 -> [_]
          shift-right: [w280] -> _
          shift-left: w264 -> [w279]
          tunnel: w273 -> [w276]
          stop <- w282 continue-if-true
          # "Updates wavelength\nwhile moving to new one"
          n148 = call "Query Motor Position (TRIAX).vi"("error in (no error)"=w279, "VISA resource name"=w276) -> ("error out"=w278:errorcluster, "wavelength"=w277:dbl[unit])  [unwired: 7 in, 1 out]
          n149 = Wait on Occurrence(1:FALSE ("ignore previous (T)"), 2:w284, 3:10 ("ms timeout (-1)")) -> (0:w282:bool)
          n150 = local write "Center Wavelength"(w277) -> ()
          n151 = call <vilib>:"Clear Errors.vi"("error in (no error)"=w278) -> ("error out"=w280:errorcluster)  [unwired: 5 in, 1 out]
        }
        n152 = Bundle By Name(cluster=w272, "JYCCDLib.IJYCCDReqd"=w271, "JYMONOLib.IJYMonoReqd"=w270) -> (w262:refnum<class "Synapse CCD.lvclass">)
      }
      event "Set CCD": Value Change {
        # "ADC Query Method is broken\n\nKeep track of it manually in \nmember data"
        n153 = event-data() -> ()  [unwired: 1 in, 5 out]
        n154 = local write "where am i?"("step1" ("where am i?")) -> ()
        n155 = Unbundle By Name(w314) -> ("JYCCDLib.IJYCCDReqd"=w309:refnum<k7>, "Areas"=w317:T2)
        n156 = Index Array(array=w317, index (col)=0 ("index (row)")) -> (element=w316:i32[])  [unwired: 1 in]
        n157 = Array Size(array=w316) -> (size(s)=w315:i32)
        n158 = flat-sequence {
          tunnel: w315 -> [w336]
          tunnel: w317 -> [w335]
          tunnel: w309 -> [w329]
          tunnel: w322 -> [w330]
          tunnel: [w333] -> w321
          tunnel: w314 -> [w332]
          tunnel: [w324] -> w318
          tunnel: w321 -> [w342]
          tunnel: [w342] -> w319
          tunnel: [w338] -> w312
          tunnel: w318 -> [w341]
          tunnel: w319 -> [w349]
          tunnel: [w348] -> w311
          tunnel: [w353] -> w313
          tunnel: w311 -> [w353]
          frame #0 {
            w327 = 1 items=["JYMCD_ACQ_FORMAT_IMAGE", "JYMCD_ACQ_FORMAT_SCAN"] ("Acquisition type")
            n159 = local write "where am i?"("step2" ("where am i?")) -> ()
            n160 = local read "Integration time"() -> (w334:dbl[unit])
            n161 = local read "GAIN"() -> (w328:u16)
            n162 = local read "ADC"() -> (w325:u16)
            n163 = node(w334) -> (w326:dbl)
            n164 = call "Setup CCD.vi"("IJYCCDReqd In"=w329, "Integration time(ms)"=w326, "Select ADC"=w325, "Gain"=w328, "Acquisition type"=w327, "error in (no error)"=w330, "numAreas"=w336, "areas :"=w335) -> ("IJYCCDReqd Out"=w331:refnum<k7>, "error out"=w333:errorcluster)  [unwired: 5 in, 1 out]
            n165 = Bundle By Name(cluster=w332, "ADC"=w325, "JYCCDLib.IJYCCDReqd"=w331) -> (w324:refnum<class "Synapse CCD.lvclass">)
          }
          frame #1 {
            n166 = local write "where am i?"("step3" ("where am i?")) -> ()
            n167 = local read "Time Between Acq. (ms)"() -> (w343:u32)
            n168 = local read "Cosmic Ray\nRemoval?"() -> (w339:bool)
            n169 = local read "Dark Subtract?"() -> (w345:bool)
            n170 = local read "# to Average"() -> (w344:u32)
            n171 = local read "Averaging?"() -> (w340:bool)
            n172 = call "Setup Multi Acq.vi"("# of Scans"=w344, "Time Between Acq (ms)"=w343, "Cosmic Ray Removal?"=w339, "Averaging?"=w340, "Dark Subtract?"=w345, "Synapse CCD.lvclass In"=w341) -> ("Synapse CCD.lvclass Out"=w338:refnum<class "Synapse CCD.lvclass">)  [unwired: 5 in]
          }
          frame #2 {
            n173 = Wait (ms)(milliseconds to wait=u32 100) -> ()  [unwired: 1 out]
            n174 = local write "where am i?"("step4" ("where am i?")) -> ()
            n175 = property on="Populate Fields with Member Data" class="Bool (strict)"(error in=w349, "Val(Sgnl)"=TRUE) -> (error out=w348:errorcluster)  [unwired: 1 in, 1 out]
          }
          frame #3 {
            n176 = local write "Set CCD"(FALSE ("Set CCD")) -> ()
            n177 = local write "where am i?"("step5" ("where am i?")) -> ()
          }
        }
      }
      event "Take Spectrum": Value Change {
        n178 = event-data() -> ()  [unwired: 1 in, 5 out]
        n179 = Bundle By Name(cluster=w359, "Raster Scan?"=FALSE ("Raster Scan.Raster Scan?")) -> (w358:refnum<class "Synapse CCD.lvclass">)
        n180 = flat-sequence {
          tunnel: [w385] -> w362
          tunnel: [w384] -> w361
          tunnel: [w381] -> w364
          tunnel: w360 -> [w379]
          tunnel: w358 -> [w376]
          tunnel: w362 -> [w388]
          tunnel: w361 -> [w390]
          tunnel: [w387] -> w363
          tunnel: [w389] -> w355
          tunnel: [w386] -> w371
          frame #0 {
            n181 = local read "Bin width (nm)\n(scan resolution)"() -> (w382:dbl[unit])
            n182 = node(w382) -> (w383:dbl)
            n183 = call "Multi-Acq.vi"("error in"=w379, "Synapse CCD.lvclass In"=w376) -> ("error out"=w378:errorcluster, "Synapse CCD.lvclass Out"=w377:refnum<class "Synapse CCD.lvclass">)  [unwired: 7 in, 1 out]
            n184 = call "Multi Data Processor.vi"("error in (no error)"=w378, "Step Size"=w383, "Synapse CCD.lvclass In"=w377) -> ("error out"=w384:errorcluster, "Processed Spectrum"=w381:cluster{"Ramp Pattern":dbl[], "X array":dbl[]}[], "Synapse CCD.lvclass Out"=w385:refnum<class "Synapse CCD.lvclass">, "Cosmic Ray Location(s)"=w380:string)  [unwired: 4 in, 1 out]
            n185 = local write "Cosmic Ray Locations"(w380) -> ()
          }
          frame #1 {
            n186 = local write "Take Spectrum"(FALSE ("Take Spectra")) -> ()
            n187 = call "Get Axis.vi"("error in (no error)"=w390, "Synapse CCD.lvclass in"=w388) -> ("error out"=w389:errorcluster, "Array of Wavelengths"=w386:dbl[], "Synapse CCD.lvclass out"=w387:refnum<class "Synapse CCD.lvclass">)  [unwired: 7 in]
          }
        }
        n188 = Index Array(array=w364, index=0) -> (element=w367:cluster{"Ramp Pattern":dbl[], "X array":dbl[]})
        n189 = Unbundle By Name(w367) -> ("X array"=w366:dbl[])
        n190 = Array Max & Min(array=w366) -> (max value=→"Max value of last snapshot":dbl)  [unwired: 3 out]
        n191 = Unbundle By Name(w363) -> ("Raw Data"=w375:i32[][])
        n192 = property on="Populate Fields with Member Data" class="Bool (strict)"(error in=w355, "Val(Sgnl)"=TRUE ("Value (Signaling)")) -> (error out=w354:errorcluster)  [unwired: 1 in, 1 out]
        n193 = Index Array(array=w375) -> (element #1=w374:i32[], element #2=w370:i32[])  [unwired: 4 in]
        n194 = Bundle("Array of Wavelengths"=w371, "Raw Data"=w374) -> (w373:T10)  [unwired: 1 in]
        n195 = Bundle("Array of Wavelengths"=w371, "Raw Data"=w370) -> (w369:T10)  [unwired: 1 in]
        n196 = Build Array(w373, w369) -> (→"UnProcessed Spectra":T1)
        "Spectrum" <- w364
      }
      event "estimate laser Pulse?": Value Change {
        n197 = event-data() -> ()  [unwired: 1 in, 6 out]
        n198 = flat-sequence {
          tunnel: [w395] -> w394
          tunnel: w393 -> [w395]
          frame #0 {
            n199 = Wait (ms)(milliseconds to wait=u32 200) -> ()  [unwired: 1 out]
            n200 = call "LaserPulseCalc.vi"() -> ("Pulse width FWHM"=w397:dbl[unit])  [unwired: 4 in]
            n201 = local write "laser Pulse"(w397) -> ()
          }
          frame #1 {
            n202 = local write "estimate laser Pulse?"(FALSE ("estimate laser Pulse?")) -> ()
          }
        }
      }
      event "image mode": Value Change {
        n203 = event-data() -> ()  [unwired: 1 in, 6 out]
        n204 = vi-ref "Image mode.vi"() -> (w400:refnum<vi>)
        n205 = call "Application Launcher.vi"("Toggle?"="image mode", "VI reference"=w400) -> ()  [unwired: 1 in, 9 out]
      }
      event "stop": Value Change {
        n206 = event-data() -> ()  [unwired: 1 in, 5 out]
      }
    }
  }
  n207 = call-dynamic "_Destroy.vi"("error in (no error)"=w17, "Synapse CCD in"=w18) -> ("error out"=→"error out":errorcluster)  [unwired: 9 in]
